vi "RdPara.vi"(8 "error in":errorcluster caption="错误输入", 9 "XLSName":string="设备型号AB", 11 "PathIn":path=path "E:/桌面/小程序/M项目条码生成1.0") -> (0 "error out":errorcluster caption="错误输出", 3 "参数配置":T1)   [LabVIEW 2013]
uses:
  ParaConfig.ctl
  Global.vi
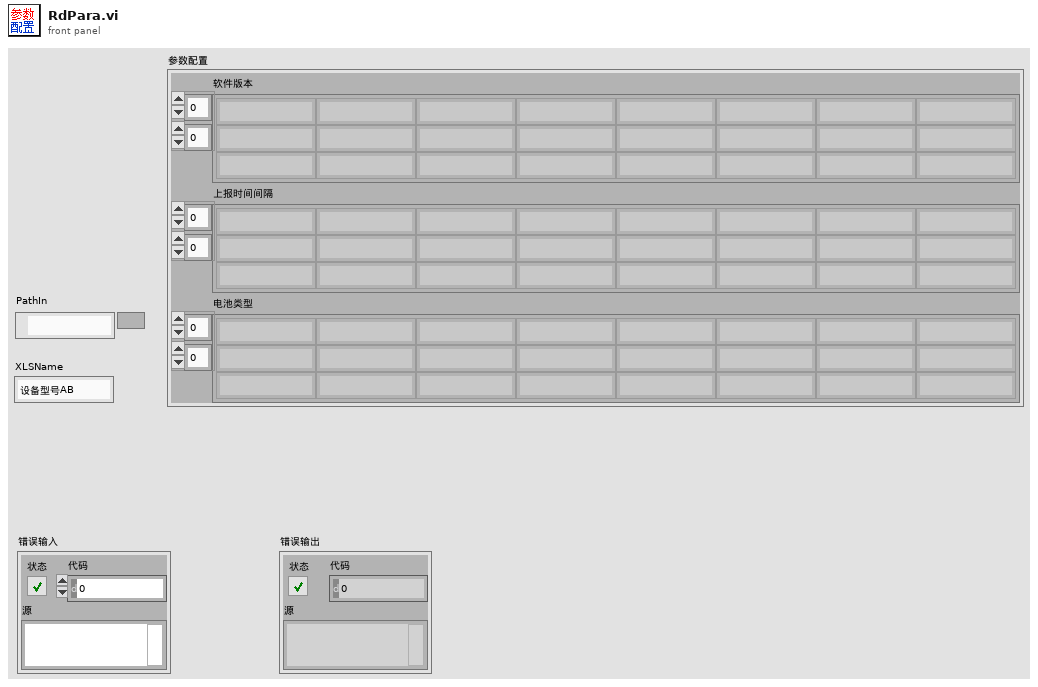
[diagram p1: front panel]
types:
  T1 = typedef "ParaConfig.ctl" = cluster{"软件版本":string[][], "上报时间间隔":string[][], "电池类型":string[][]}
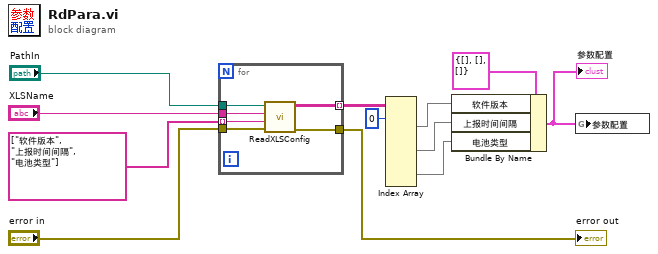
[diagram p0: block diagram]
diagram:
  n1 = for {
    tunnel: "XLSName" -> [w18]
    tunnel: "PathIn" -> [w17]
    tunnel: string[] ["软件版本", "上报时间间隔", "电池类型"] -> [w16] mode=indexing
    tunnel: [w15] -> w8 mode=indexing
    tunnel: "error in" -> [w14]
    tunnel: [w13] -> w1
    n2 = call "ReadXLSConfig.vi"("error in"=w14, "pagename"=w16, "XLSName"=w18, "PathIn"=w17) -> ("error out"=w13:errorcluster, "Data"=w15:string[][])  [unwired: 6 in]
  }
  "error out" <- w1
  n3 = Index Array(array=w8, index (dim 0) #1=0 ("索引 (页)")) -> (element #1=w4:string[][], element #2=w3:string[][], element #3=w2:string[][])  [unwired: 8 in]
  n4 = Bundle By Name(cluster=T1 {"软件版本"=[], "上报时间间隔"=[], "电池类型"=[]} ("参数配置"), "软件版本"=w4, "上报时间间隔"=w3, "电池类型"=w2) -> (w5:T1)
  "参数配置" <- w5
  n5 = global write "Global.vi" "参数配置"(w5) -> ()
